vi "BigIntToHexString-Octect.vi"(1 "a":cluster{"Boolean":bool, "Array":u64[]}) -> (0 "Hex string":string)   [LabVIEW 2023]
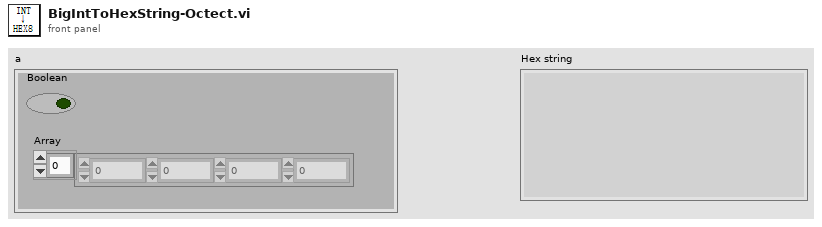
[diagram p1: front panel]
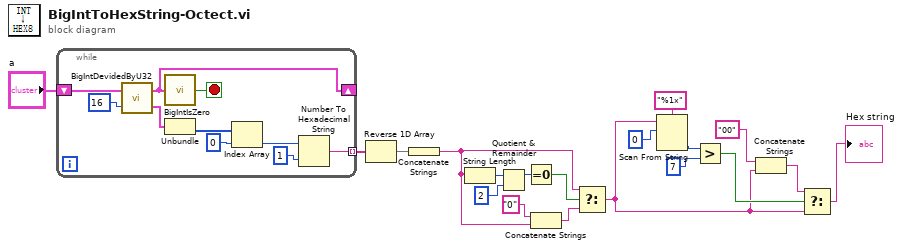
[diagram p0: block diagram]
diagram:
  n1 = while {
    shift-right: [w20] -> _
    shift-left: "a" -> [w29]
    tunnel: [w21] -> w18 mode=indexing
    stop <- w27 stop-if-true
    n2 = call "BigIntDevidedByU32.vi"("b (<1e9)"=u64 16, "a"=w29) -> ("a % b"=w26:cluster{"Boolean":bool, "Array":u64[]}, "a / b"=w20:cluster{"Boolean":bool, "Array":u64[]})
    n3 = call "BigIntIsZero.vi"("a"=w20) -> ("a = 0"=w27:bool)
    n4 = Unbundle(w26) -> ("Array"=w25:u64[])  [unwired: 1 out]
    n5 = Index Array(array=w25, index=0) -> (element=w23:u64)
    n6 = Number To Hexadecimal String(1:1, 2:w23) -> (0:w21:string)
  }
  n7 = Reverse 1D Array(array=w18) -> (reversed array=w17:string[])
  n8 = Concatenate Strings(w17) -> (w2:string)
  n9 = String Length(string=w2) -> (length=w8:i32)
  n10 = Quotient & Remainder(x=w8, y=2) -> (x-y*floor(x/y)=w6:i32)  [unwired: 1 out]
  n11 = Equal To 0?(x=w6) -> (x = 0?=w5:bool)
  n12 = Concatenate Strings("0", w2) -> (w1:string)
  n13 = Select(t=w2, s=w5, f=w1) -> (s? t:f=w4:string)
  n14 = Scan From String(format string="%1x", input string=w4, initial scan location=0) -> (output 1=w11:u32)  [unwired: 2 in, 3 out]
  n15 = Greater?(x=w11, y=u32 7) -> (0:w15:bool)
  n16 = Concatenate Strings("00", w4) -> (w13:string)
  n17 = Select(t=w13, s=w15, f=w4) -> (s? t:f=→"Hex string":string)
